vi "DB_Insert.vi"() -> ()   [LabVIEW 2020]
uses:
  <vilib>/addons/database/Connection.llb/DB Tools Open Connec (String).vi
  <vilib>/addons/database/_DB Variant To Data/Database Variant To Data.xnode
  <vilib>/addons/database/NI_Database_API.lvlib
panel:
  out "Table_ID":string[][](array[string])
  in  "Database":T1(array[cluster])=[{"Nom"="Dupont", "Prénom"="Marie", "age"=32.0, "Sexe"="F", "Métier"="Ingénieure", "Rémunération"=45000.0}, {"Nom"="Dupont", "Prénom"="Jacques", "age"=45.0, "Sexe"="H", "Métier"="Développeur", "Rémunération"=50000.0}, {"Nom"="Leroy", "Prénom"="Sophie", "age"=28.0, "Sexe"="F", "Métier"="Analyste", "Rémunération"=42000.0}, {"Nom"="Bernard", "Prénom"="Thomas", "age"=39.0, "Sexe"="H", "Métier"="Consultant", "Rémunération"=55000.0}, {"Nom"="Moreau", "Prénom"="Claire", "age"=31.0, "Sexe"="F", "Métier"="Designer", "Rémunération"=40000.0}] {"Rémunération" format="%#_g €"}
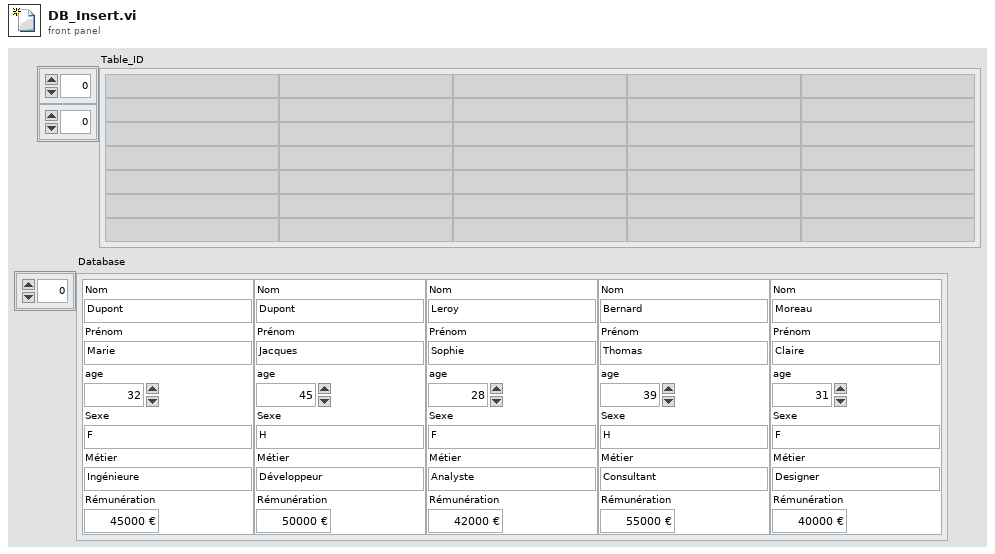
[diagram p1: front panel]
types:
  T1 = cluster{"Nom":string, "Prénom":string, "age":sgl, "Sexe":string, "Métier":string, "Rémunération":sgl}[]
  T2 = typedef "NI_Database_API.lvlib/Conn ObjectReference.ctl" = refnum<k1>
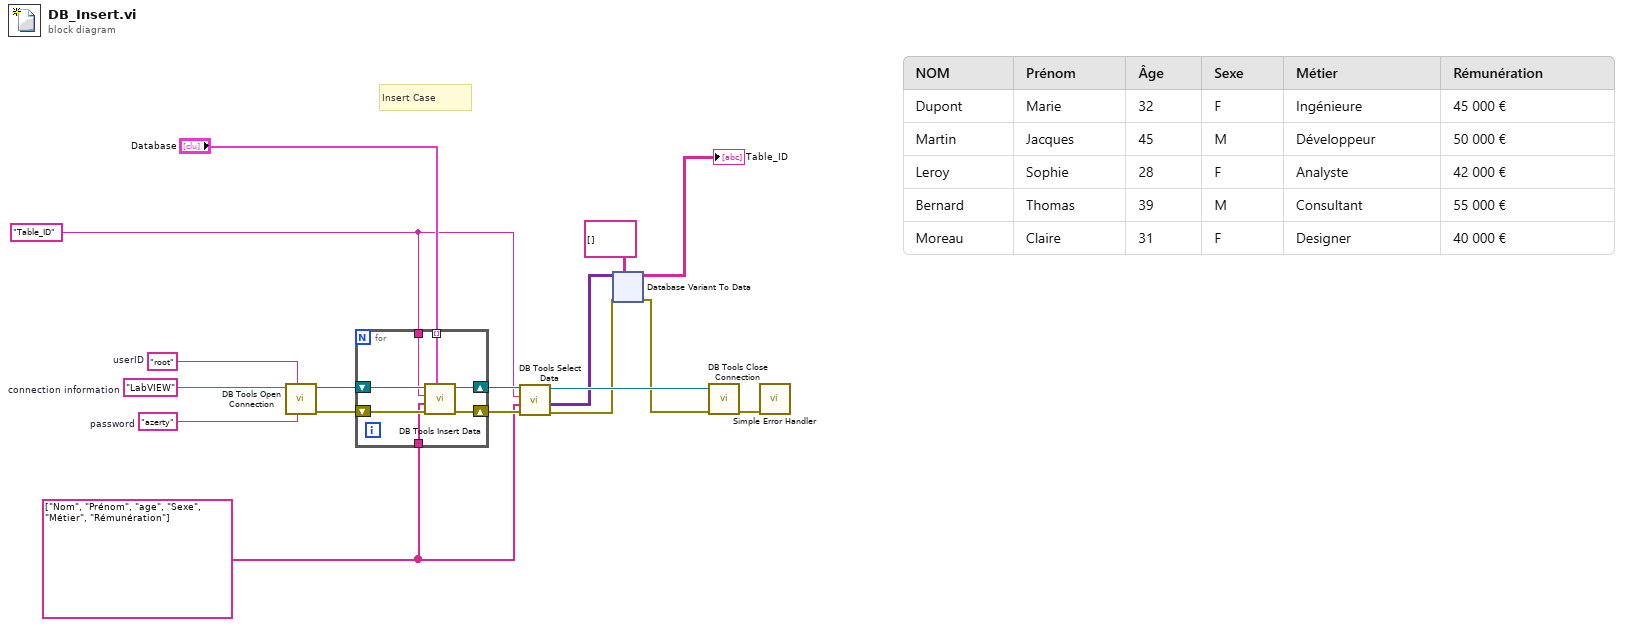
[diagram p0: block diagram]
diagram:
  w1 = "azerty"  # password
  w2 = "root"  # userID
  w9 = string[] ["Nom", "Prénom", "age", "Sexe", "Métier", "Rémunération"] ("columns")
  w10 = "Table_ID" ("table")
  w3 = "LabVIEW"  # connection information
  # "Insert Case"
  n1 = call-poly <vilib>:"DB Tools Open Connection.vi"("password"=w1, "userID"=w2, "connection information"=w3) -> ("error out"=w16:errorcluster, "connection reference"=w15:T2)  [unwired: 5 in]
  n2 = for {
    tunnel: "Database" -> [w22] mode=indexing
    tunnel: w10 -> [w19]
    tunnel: w9 -> [w18]
    shift-right: [w20] -> w12
    shift-left: w16 -> [w24]
    shift-right: [w21] -> w13
    shift-left: w15 -> [w23]
    n3 = call <vilib>:"DB Tools Insert Data.vi"("data"=w22, "error in (no error)"=w24, "columns"=w18, "table"=w19, "connection reference"=w23) -> ("error out"=w20:errorcluster, "connection reference out"=w21:T2)  [unwired: 5 in]
  }
  n4 = call <vilib>:"DB Tools Select Data.vi"("error in (no error)"=w12, "columns"=w9, "table"=w10, "connection reference"=w13) -> ("error out"=w7:errorcluster, "data"=w8:variant[][], "connection reference out"=w11:T2)  [unwired: 2 in]
  n5 = xnode "Database Variant To Data"("database variant"=w8, "error in (no error)"=w7, "type"=string[][] []) -> ("data"=→"Table_ID":string[][], "error out"=w6:errorcluster)
  n6 = call <vilib>:"DB Tools Close Connection.vi"("error in (no error)"=w6, "connection reference"=w11) -> ("error out"=w17:errorcluster)  [unwired: 5 in]
  n7 = call <vilib>:"Simple Error Handler.vi"("error in (no error)"=w17) -> ()  [unwired: 4 in, 5 out]
